vi "Condition Name.vi"(8 "error in":errorcluster, 9 "Terminals (All)":T2, 10 "Name":T1) -> (0 "error out":errorcluster)   [LabVIEW 2020, in "_Rescript.lvlib" / "Actor.lvlib" / "Actor.lvclass"]
uses:
  Actor.lvclass
  Terminals.ctl
  Name.ctl
  _Rescript.lvlib
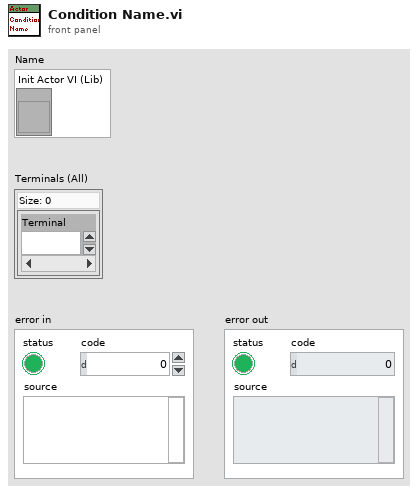
[diagram p1: front panel]
types:
  T1 = typedef "_Rescript.lvlib/Actor.lvlib/Actor.lvclass/Name.ctl" = cluster{"Init Actor VI (Lib)":refnum<vi>}
  T2 = typedef "_Rescript.lvlib/Terminals.ctl" = set{i32}
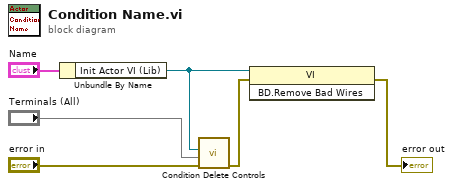
[diagram p0: block diagram]
diagram:
  n1 = Unbundle By Name("Name") -> ("Init Actor VI (Lib)"=w1:refnum<vi>)
  n2 = call "Condition Delete Controls.vi"("error in"="error in", "Terminals"="Terminals (All)", "VI"=w1) -> ("error out"=w2:errorcluster)  [unwired: 8 in]
  n3 = invoke class="VI" method="BD.Remove Bad Wires"(reference=w1, error in=w2) -> (error out=→"error out":errorcluster)  [unwired: 1 in, 2 out]
